vi "Package Dependencies.vi"(7 "Absolute Path (F)":bool, 8 "error in (no error)":errorcluster, 11 "PackageAbstract in":refnum<class "PackageAbstract.lvclass">) -> (0 "error out":errorcluster, 2 "Dependencies":T1[](array[typedef]))   [LabVIEW 2020, in "GPack.lvlib" / "PackageAbstract.lvclass"]
uses:
  PackageAbstract.lvclass
  Dependency.ctl
  Package Info.ctl
  PackageAbstract.lvclass/PackageAbstract.ctl
  Package/Package.lvclass
  GPack.lvlib
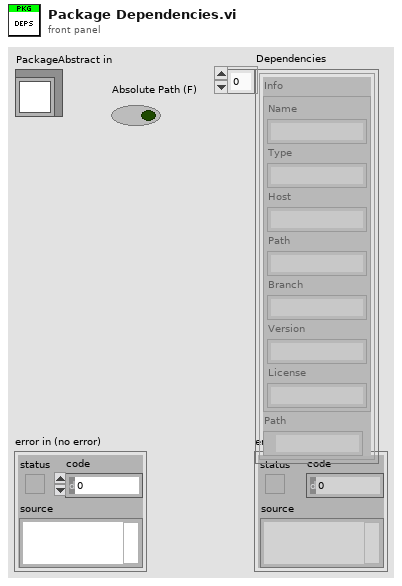
[diagram p1: front panel]
types:
  T1 = typedef "GPack.lvlib/Dependency.ctl" = cluster{"Info":T2, "Path":path}
  T2 = typedef "GPack.lvlib/Package Info.ctl" = cluster{"Name":string, "Type":string, "Host":string, "Path":string, "Branch":string, "Version":string, "License":string}
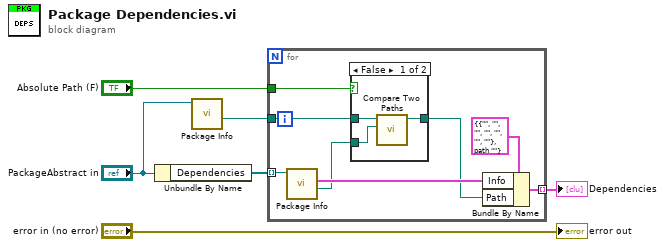
[diagram p0: block diagram]
diagram:
  n1 = Unbundle By Name("PackageAbstract in") -> ("Dependencies"=w5:refnum<class "Package.lvclass">[])
  n2 = call-dynamic "Package Info.vi"("Package in"="PackageAbstract in") -> ("Folder"=w2:path)  [unwired: 8 in, 2 out]
  n3 = for {
    tunnel: w5 -> [w14] mode=indexing
    tunnel: [w11] -> w4 mode=indexing
    tunnel: w2 -> [w10]
    tunnel: "Absolute Path (F)" -> [w7]
    n4 = call-dynamic "Package Info.vi"("Package in"=w14) -> ("Folder"=w9:path, "Package Info"=w12:T2)  [unwired: 8 in, 1 out]
    n5 = case shown="False" w7 {
      tunnel: w10 -> [w17 _]
      tunnel: w9 -> [w16 w18]
      tunnel: [w15 w18] -> w8
      frame False {
        n6 = call <vilib>:"Compare Two Paths.vi"("Path 2"=w16, "Path 1"=w17) -> ("Relative Path from 1 to 2"=w15:path)  [unwired: 6 in, 3 out]
      }
      frame True {
      }
    }
    n7 = Bundle By Name(cluster=T1 {"Info"={"Name"="", "Type"="", "Host"="", "Path"="", "Branch"="", "Version"="", "License"=""}, "Path"=path ""} ("Dependency"), "Info"=w12, "Path"=w8) -> (w11:T1)
  }
  "Dependencies" <- w4
  "error out" <- "error in (no error)"
